vi "All Channels.vi"(8 "error in (no error)":errorcluster, 11 "Group in":refnum<class "Group DBL.lvclass">) -> (0 "error out":errorcluster, 2 "All Channels":refnum<class "Channel DBL.lvclass">[](array[class]), 3 "Group out":refnum<class "Group DBL.lvclass">)   [LabVIEW 2020, in "Vecto.lvlib" / "Group DBL.lvclass"]
uses:
  Group DBL.lvclass
  C:/dev/lv20CE/relink/lv-vecto/Vecto/Group/Group.lvclass
  Channel DBL/Channel DBL.lvclass
  Group/Group.lvclass/Group.ctl
  Channel DBL/Channel DBL.lvclass/Channel DBL.ctl
  Group Config/Get Channels.vi
  Group/Group.lvclass
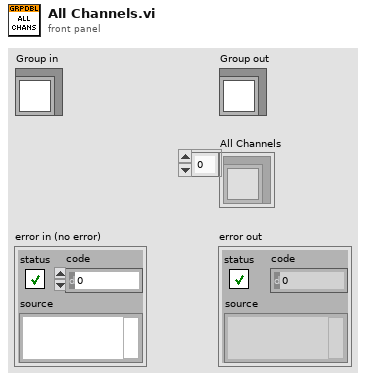
[diagram p1: front panel]
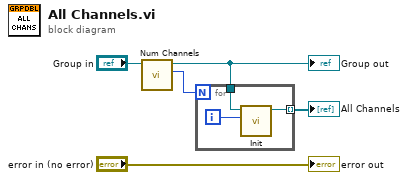
[diagram p0: block diagram]
diagram:
  n1 = call "Num Channels.vi"("GroupAbstract in"="Group in") -> ("Num Channels"=w1:i32, "GroupAbstract out"=w2:refnum<class "Group DBL.lvclass">)  [unwired: 8 in, 1 out]
  "Group out" <- w2
  n2 = for {
    N: w1 -> [_]
    tunnel: w2 -> [w7]
    tunnel: [w6] -> w4 mode=indexing
    i -> [w8]
    n3 = call "Init.vi"("Channel Index"=w8, "Group"=w7) -> ("Channel out"=w6:refnum<class "Channel DBL.lvclass">)  [unwired: 8 in, 1 out]
  }
  "All Channels" <- w4
  "error out" <- "error in (no error)"
